vi "Configure Measurement Characteristics.vi"(5 "Autozero Mode (2: Autozero Auto)":i32(ring)=2 items=["Autozero Off", "Autozero Once", "Autozero Auto"], 6 "Measurement Interval (0 S)":dbl, 7 "Measurement Aperture (1)":dbl=1.0, 8 "error in (no error)":errorcluster, 9 "Measurement Count (1)":i32=1, 10 "Source Measure Unit Channel (0: Channel A)":i32(ring) items=["Channel A", "Channel B"], 11 "VISA resource name":refnum<visa-resource-name>) -> (0 "error out":errorcluster, 3 "VISA resource name out":refnum<visa-resource-name>)   [LabVIEW 2015, in "Keithley 2600 Series.lvlib"]
doc: "Configures the basic settings for the measurement."
uses:
  Keithley 2600 Series.lvlib
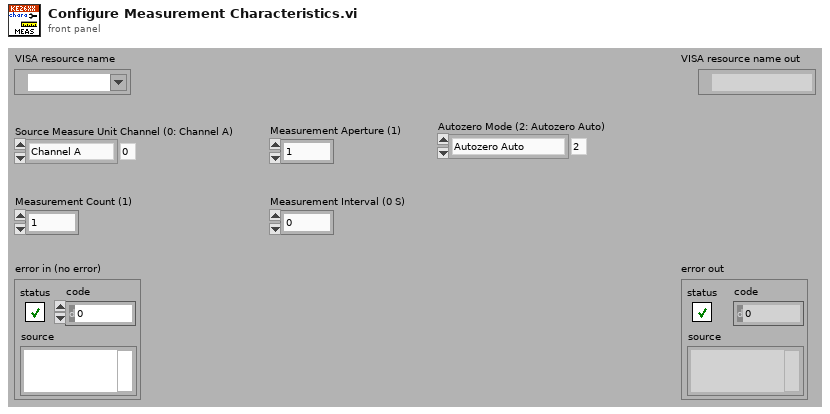
[diagram p1: front panel]
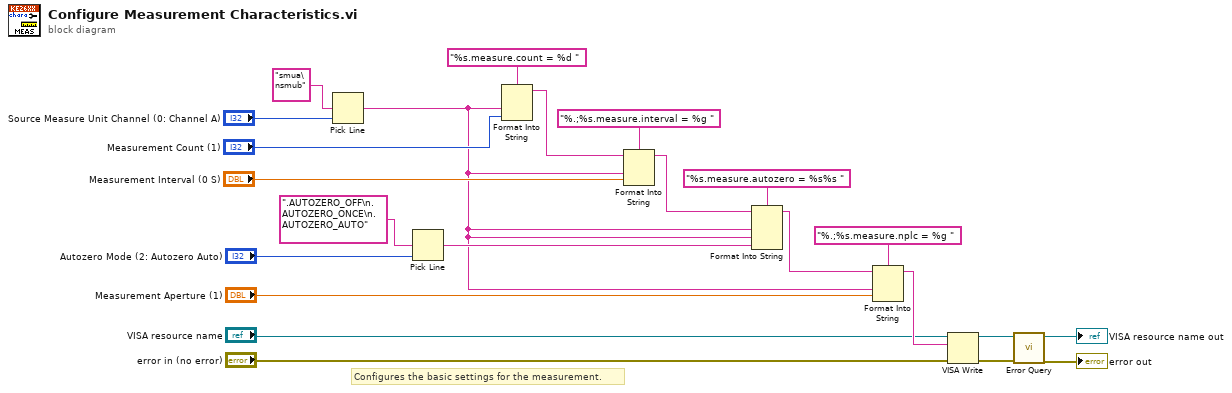
[diagram p0: block diagram]
diagram:
  # "Configures the basic settings for the measurement."
  n1 = Pick Line(multi-line string="smua\nsmub", line index="Source Measure Unit Channel (0: Channel A)") -> (output string=w1:string)  [unwired: 1 in]
  n2 = Pick Line(multi-line string=".AUTOZERO_OFF\n.AUTOZERO_ONCE\n.AUTOZERO_AUTO", line index="Autozero Mode (2: Autozero Auto)") -> (output string=w2:string)  [unwired: 1 in]
  n3 = Format Into String(format string="%s.measure.count = %d ", w1, "Measurement Count (1)") -> (resulting string=w21:string)  [unwired: 2 in, 1 out]
  n4 = Format Into String(format string="%.;%s.measure.interval = %g ", initial string=w21, w1, "Measurement Interval (0 S)") -> (resulting string=w18:string)  [unwired: 1 in, 1 out]
  n5 = Format Into String(format string="%s.measure.autozero = %s%s ", initial string=w18, w1, w1, w2) -> (resulting string=w16:string)  [unwired: 1 in, 1 out]
  n6 = Format Into String(format string="%.;%s.measure.nplc = %g ", initial string=w16, w1, "Measurement Aperture (1)") -> (resulting string=w13:string)  [unwired: 1 in, 1 out]
  n7 = VISA Write(VISA resource name="VISA resource name", write buffer=w13, error in (no error)="error in (no error)") -> (VISA resource name out=w10:refnum<visa-resource-name>, error out=w9:errorcluster)  [unwired: 1 out]
  n8 = call "Error Query.vi"("error in (no error)"=w9, "VISA resource name"=w10) -> ("error out"=→"error out":errorcluster, "VISA resource name out"=→"VISA resource name out":refnum<visa-resource-name>)  [unwired: 6 in, 2 out]
